vi "Setup subWorker - DataSave Worker.vi"(8 "error in":errorcluster, 11 "DAQ Worker in":refnum<class "DAQ Worker.lvclass">) -> (0 "error out":errorcluster, 3 "DAQ Worker out":refnum<class "DAQ Worker.lvclass">)   [LabVIEW 2020, in "DAQ Worker.lvclass"]
doc: "This VI sets up the framework parameters of a statically-linked subWorker."
uses:
  DAQ Worker.lvclass
  DAQ Worker.lvclass/DAQ Worker.ctl
  DataSave Worker/DataSave Worker.lvclass
  C:/Program Files (x86)/National Instruments/LabVIEW 2020/vi.lib/addons/_Workers/Library/Classes/Worker/Worker.lvclass
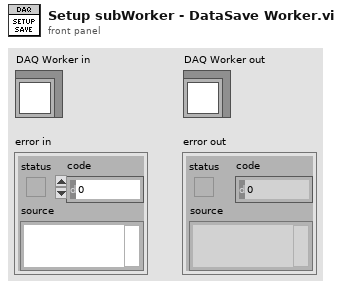
[diagram p1: front panel]
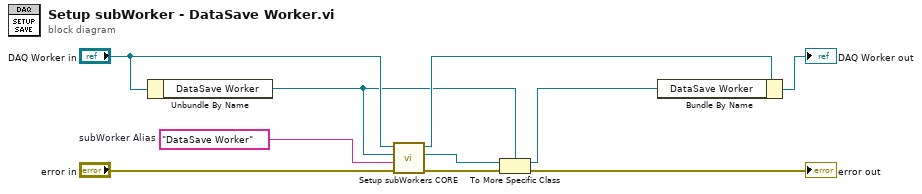
[diagram p0: block diagram]
diagram:
  w6 = "DataSave Worker"  # subWorker Alias
  n1 = Unbundle By Name("DAQ Worker in") -> ("DataSave Worker"=w3:refnum<class "DataSave Worker.lvclass">)
  n2 = call-dynamic "Setup subWorkers CORE.vi"("error in"="error in", "subWorker Alias"=w6, "subWorker"=w3, "Worker"="DAQ Worker in") -> ("error out"=w5:errorcluster, "subWorker out"=w1:refnum<class "Worker.lvclass">, "Worker out"=w8:refnum<class "DAQ Worker.lvclass">)  [unwired: 5 in]
  n3 = To More Specific Class(target class=w3, reference=w1, error in=w5) -> (specific class reference=w2:refnum<class "DataSave Worker.lvclass">, error out=→"error out":errorcluster)
  n4 = Bundle By Name(cluster=w8, "DataSave Worker"=w2) -> (→"DAQ Worker out":refnum<class "DAQ Worker.lvclass">)
